vi "GetDataVal.vi"(8 "error in (no error)":errorcluster, 10 "Name":string, 11 "ExpData in":refnum<class "ExpData.lvclass">) -> (0 "error out":errorcluster, 2 "Data":dbl[][](array[numeric]), 3 "ExpData out":refnum<class "ExpData.lvclass">, 4 "ColHeaders":string[](array[string]))   [LabVIEW 2016, in "ExpData.lvclass"]
uses:
  ExpData.lvclass
  ExpData.lvclass/ExpData.ctl
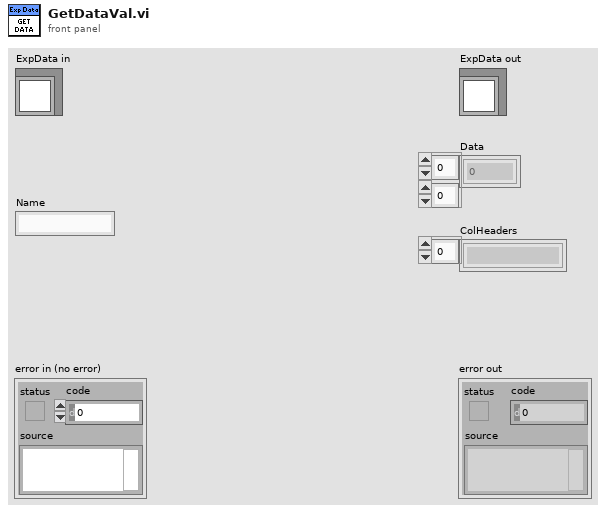
[diagram p1: front panel]
types:
  T1 = typedef "ExpData.lvclass/ColHeader.ctl" = cluster{"Name":string, "Index":i32, "Size":i32}
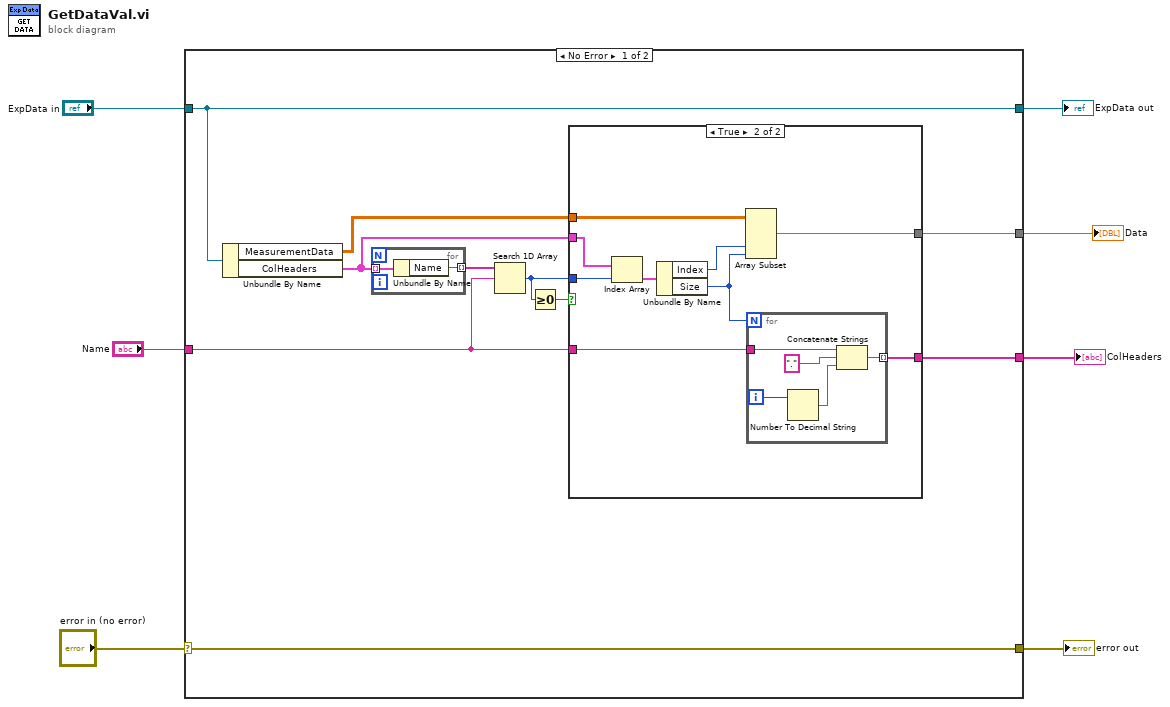
[diagram p0: block diagram]
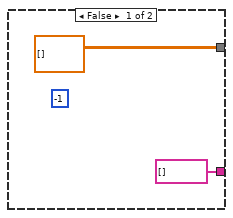
[diagram p2: hidden frame]
diagram:
  n1 = case shown="No Error" "error in (no error)" {
    selector: "error in (no error)" -> [w17 w37]
    tunnel: [w17 w37] -> w6
    tunnel: [w16 w36] -> w4
    tunnel: "ExpData in" -> [w16 w36]
    tunnel: [w10 _] -> w3
    tunnel: [w9 _] -> w2
    tunnel: "Name" -> [w8 _]
    frame No Error {
      n2 = Unbundle By Name(w16) -> ("MeasurementData"=w12:dbl[][], "ColHeaders"=w11:T1[])
      n3 = for {
        tunnel: w11 -> [w35] mode=indexing
        tunnel: [w34] -> w15 mode=indexing
        n4 = Unbundle By Name(w35) -> ("Name"=w34:string)
      }
      n5 = Search 1D Array(1D array=w15, element=w8) -> (index of element=w13:i32)  [unwired: 1 in]
      n6 = Greater Or Equal To 0?(x=w13) -> (x >= 0?=w14:bool)
      n7 = case shown="True" w14 {
        tunnel: w13 -> [_ w28]
        tunnel: w12 -> [_ w25]
        tunnel: w11 -> [_ w27]
        tunnel: [dbl[][] [] w24] -> w10
        tunnel: w8 -> [_ w21]
        tunnel: [string[] [] w20] -> w9
        frame False {
          (unwired) -1
        }
        frame True {
          n8 = Index Array(array=w27, index=w28) -> (element=w26:T1)
          n9 = Unbundle By Name(w26) -> ("Index"=w23:i32, "Size"=w22:i32)
          n10 = Array Subset(array=w25, index (col)=w23, length (col)=w22) -> (w24:dbl[][])  [unwired: 2 in]
          n11 = for {
            N: w22 -> [_]
            tunnel: w21 -> [w33]
            tunnel: [w29] -> w20 mode=indexing
            i -> [w31]
            n12 = Number To Decimal String(number=w31) -> (decimal integer string=w30:string)  [unwired: 1 in]
            n13 = Concatenate Strings(w33, "." ("string"), w30) -> (w29:string)
          }
        }
      }
    }
    frame Error {
    }
  }
  "error out" <- w6
  "ExpData out" <- w4
  "Data" <- w3
  "ColHeaders" <- w2
